vi "Main.vi"() -> ()   [LabVIEW 2022 SP3]
doc: "Use this template to build a simple state machine design pattern. Each state executes code and determines which state to transition to."
uses:
  controls/UI Data.ctl
  controls/State.ctl
  <vilib>/Utility/file.llb/Write Delimited Spreadsheet (string).vi
  <vilib>/Analysis/NI_AALBase.lvlib
panel:
  out "Zmerene vysledky":string[][](table)=[["0", "10000", "99998", "0", "99920", "0"], ["0", "0", "0", "0", "0", "0"], ["2", "10000", "99998", "0", "99920", "0"], ["0", "0", "0", "0", "0", "0"], ["0", "0", "0", "0", "0", "0"]]
  in  "Nazev souboru k ulozeni":path=path "data.txt"
  in  "Generator read error":bool
  in  "Counter read error":bool
  in  "Osciloscope read error":bool
  out "Terminal":string="RIGOL TECHNOLOGIES,DS2102A,DS2D271700283,00.03.06\nHEWLETT-PACKARD,53131A,0,3427\nAgilent Technologies,33220A,MY43002402,1.05-1.05-22-1\n+9.999795427E+004\n9.992007e+04\n+9.999795443E+004\n9.992007e+04\n+9.999795356E+004\n9.992007e+04\n+9.999795499E+004\n9.992007e+04\n+9.999795703E+004\n9.992007e+04\n+9.999795620E+004\n9.992007e+04\n"
  in  "Stop":bool
  in  "Generator source":refnum<visa-resource-name>="USB0::0x0957::0x0407::MY43002402::INSTR"
  in  "Counter source":refnum<visa-resource-name>="GPIB0::15::INSTR"
  in  "Osciloscope source":refnum<visa-resource-name>="osc"
  out "Mereni":bool
  in  "Start":bool
  in  "Nastaveni citace":T1
  in  "Pocet opakovani":u8=3 min=1 max=20
  in  "Kalibracni body":T2(array[cluster])=[{"Kmitocet"=enum."100 kHz", "Vrms (V)"=0.6}, {"Kmitocet"=enum."prazdne", "Vrms (V)"=0.6}, {"Kmitocet"=enum."100 kHz", "Vrms (V)"=2.0}, {"Kmitocet"=enum."prazdne", "Vrms (V)"=1.0}, {"Kmitocet"=enum."prazdne", "Vrms (V)"=0.6}] {"Vrms (V)" min=0.014 max=2.83}
  in  "Data":T3={"Oscilosope source"="", "Counter source"="", "Generator source"="", "Measuring?"=FALSE, "j(sample)"=0, "i(point)"=0, "Kalibracni body"=[], "Pocet opakovani"=1, "Nastaveni citace"={"Vazba"=enum."DC", "Vstupni impedance"=enum."1 MOhm", "Filtr 100 kHz"=FALSE}, "Config delay counter"=0, "GlobalState"=enum."WAITING", "Terminal"="", "namerene hodnoty osciloskop"=[], "namerene hodnoty citac"=[], "nejistoty osciloskop"=[], "nejistoty citac"=[], "vysledek citac"=[], "vysledek osciloskop"=[], "tabulka"=[]} {"Pocet opakovani" min=1 max=20}
  in  "Exit":bool
  # "Komunikace s mericimi pristroji"
  # "Spousteni mereni"
  # "Indikace stavu"
  # "Nastaveni mereni"
  # "Ne"
  # "Ano"
  # "Ano"
  # "Ne"
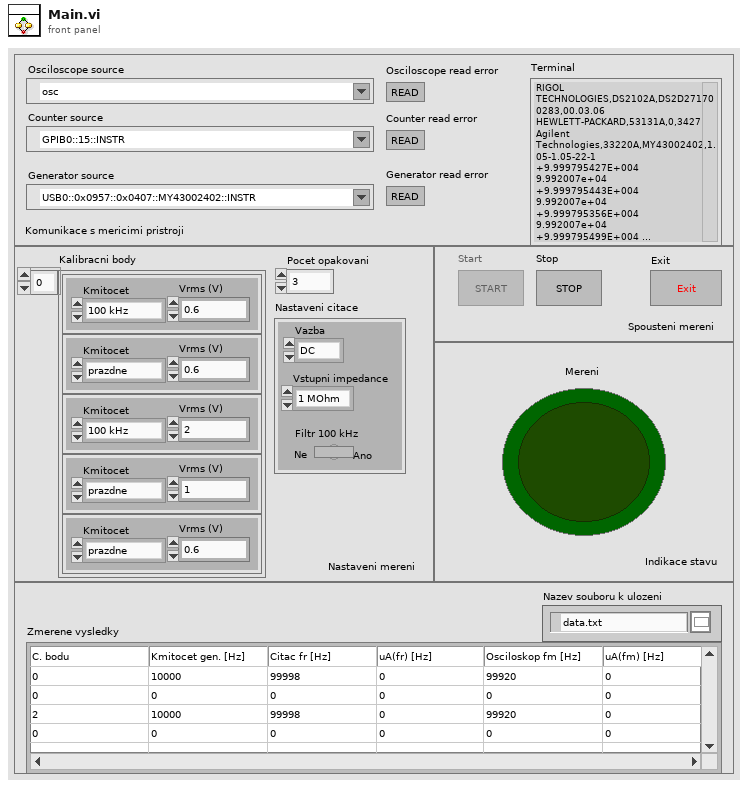
[diagram p1: front panel]
types:
  T1 = cluster{"Vazba":enum16{"DC", "AC"}, "Vstupni impedance":enum16{"1 MOhm", "50 Ohm"}, "Filtr 100 kHz":bool}
  T2 = cluster{"Kmitocet":enum16{"prazdne", "50 Hz", "1 kHz", "5 kHz", "10 kHz", "20 kHz", "50 kHz", "100 kHz"}, "Vrms (V)":dbl}[]
  T3 = typedef "UI Data.ctl" = cluster{"Oscilosope source":refnum<visa-resource-name>, "Counter source":refnum<visa-resource-name>, "Generator source":refnum<visa-resource-name>, "Measuring?":bool, "j(sample)":u8, "i(point)":u8, "Kalibracni body":cluster{"Kmitocet":enum16{"prazdne", "50 Hz", "1 kHz", "5 kHz", "10 kHz", "20 kHz", "50 kHz", "100 kHz"}, "Vrms (V)":dbl}[], "Pocet opakovani":u8, "Nastaveni citace":cluster{"Vazba":enum16{"DC", "AC"}, "Vstupni impedance":enum16{"1 MOhm", "50 Ohm"}, "Filtr 100 kHz":bool}, "Config delay counter":u8, "GlobalState":enum16{"WAITING", "NEXT", "MEASURE"}, "Terminal":string, "namerene hodnoty osciloskop":dbl[][], "namerene hodnoty citac":dbl[][], "nejistoty osciloskop":dbl[], "nejistoty citac":dbl[], "vysledek citac":dbl[], "vysledek osciloskop":dbl[], "tabulka":string[][]}
  T4 = typedef "State.ctl" = enum16{"Initialize", "Wait for Event", "Config", "Meas", "Calculate", "End meas", "Store & update", "Exit"}
  T5 = enum8{"Enabled", "Disabled", "Disabled and Grayed Out"}
  T6 = enum16{"prazdne", "50 Hz", "1 kHz", "5 kHz", "10 kHz", "20 kHz", "50 kHz", "100 kHz"}
  T7 = cluster{"Kmitocet":enum16{"prazdne", "50 Hz", "1 kHz", "5 kHz", "10 kHz", "20 kHz", "50 kHz", "100 kHz"}, "Vrms (V)":dbl}
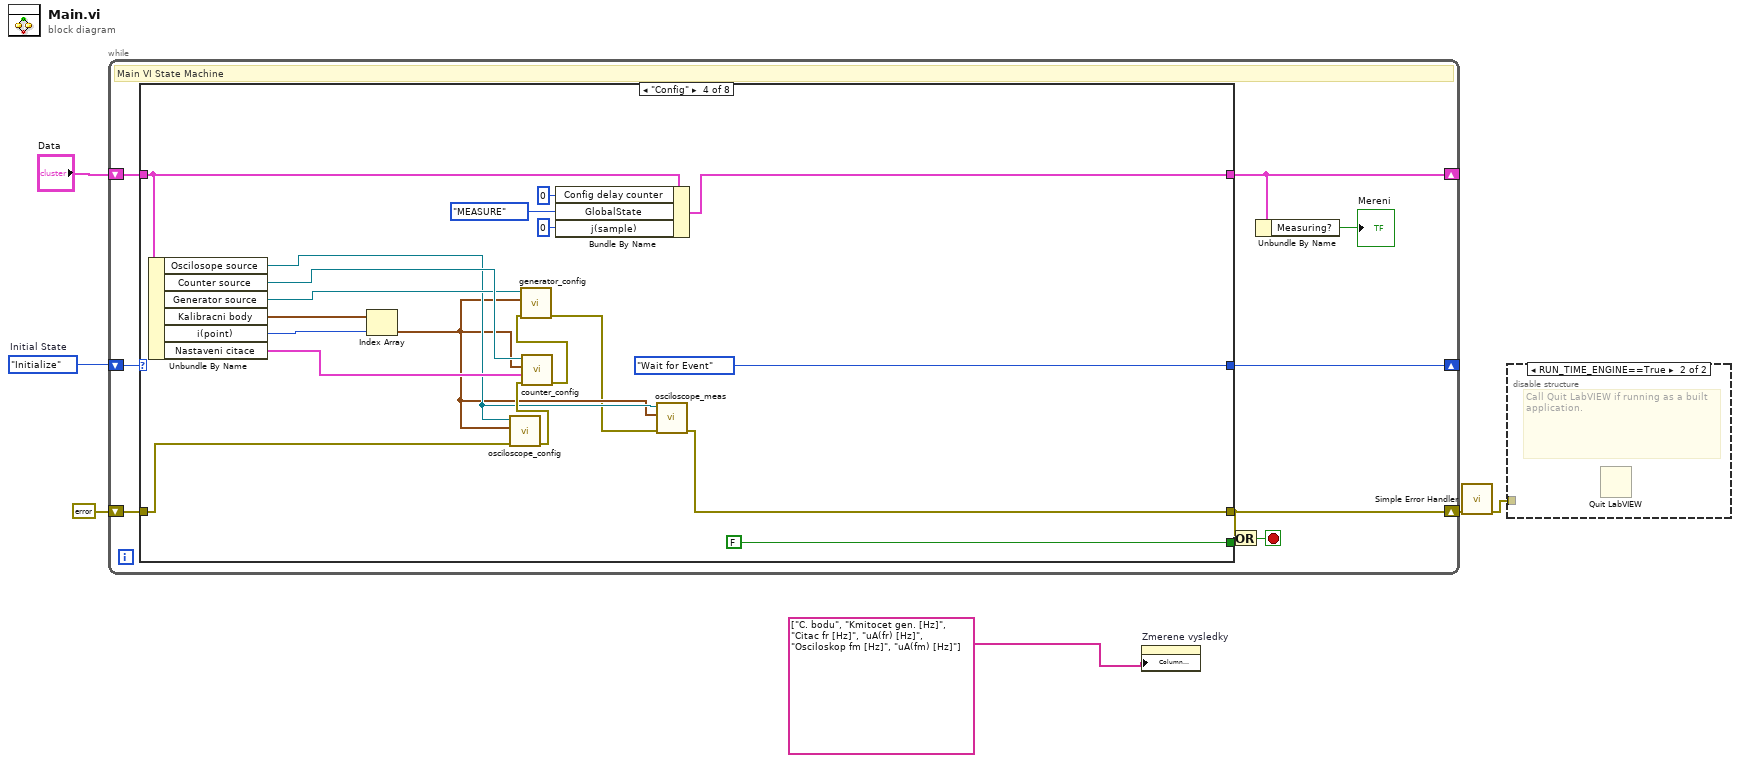
[diagram p0: block diagram]
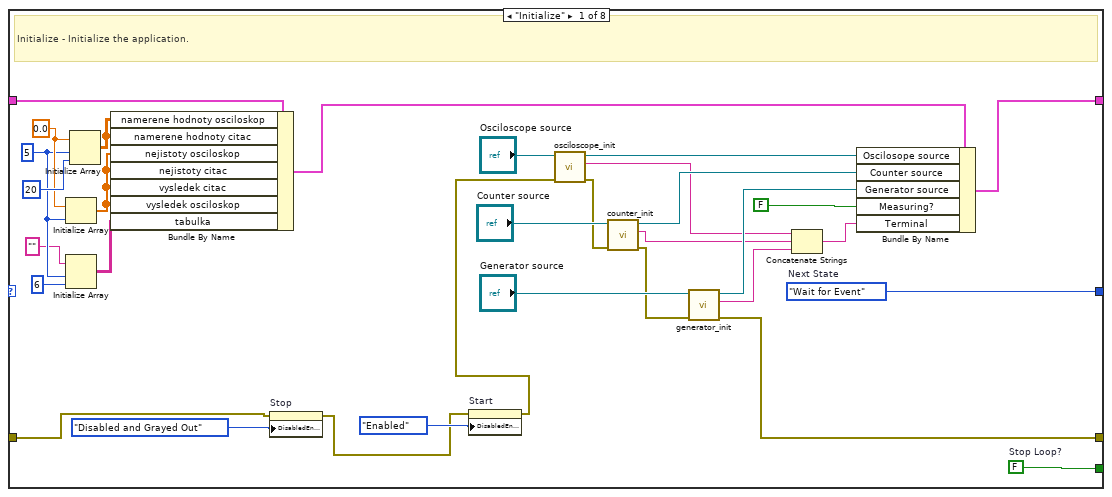
[diagram p3: hidden frame]
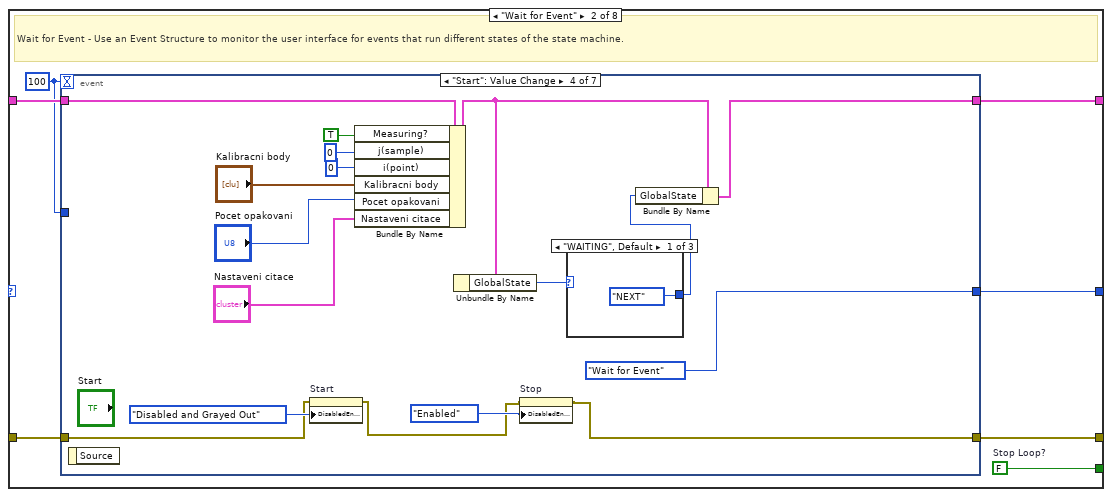
[diagram p4: hidden frame]
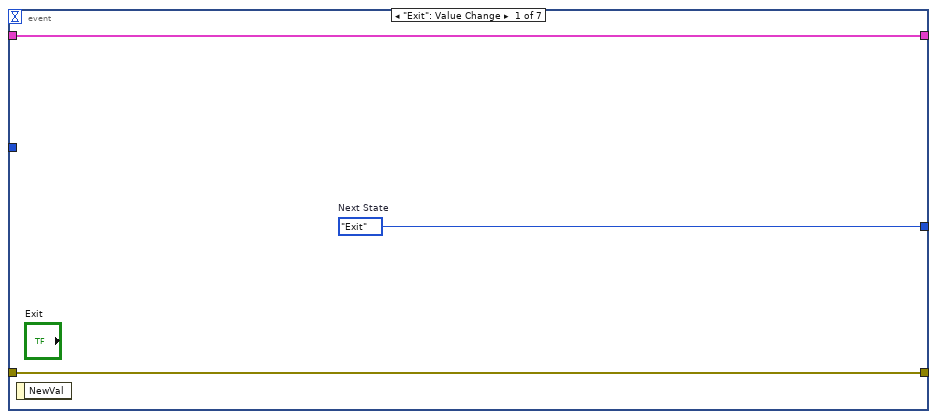
[diagram p5: hidden frame]
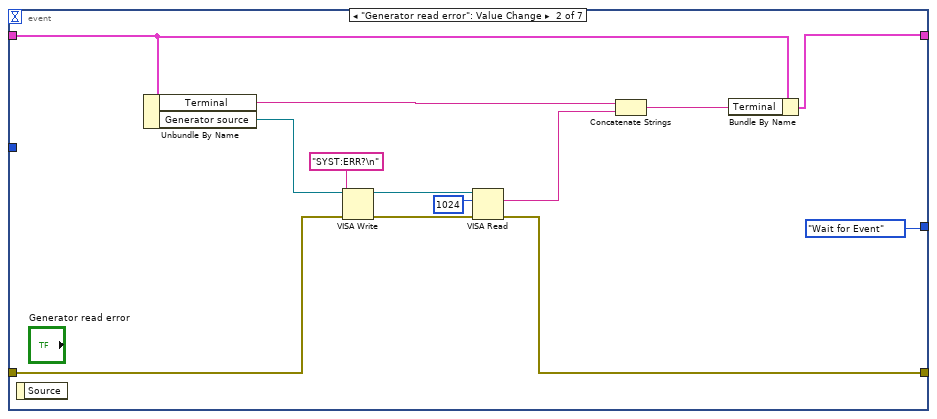
[diagram p6: hidden frame]
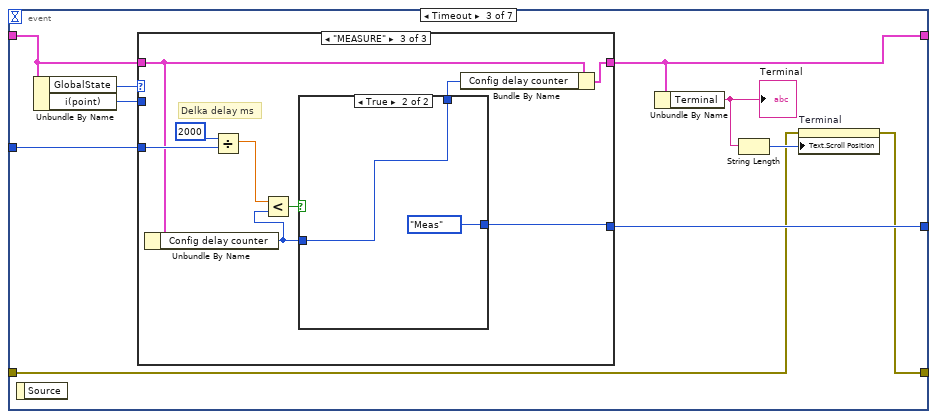
[diagram p7: hidden frame]
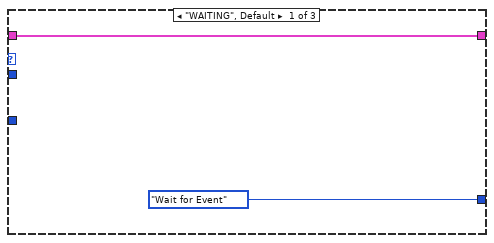
[diagram p8: hidden frame]
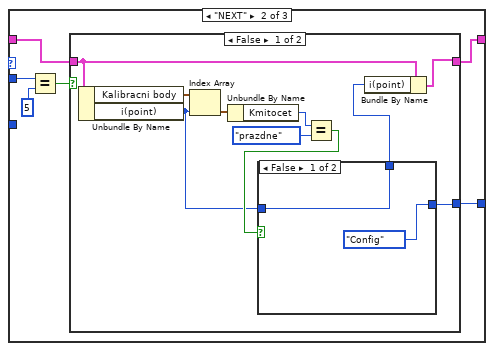
[diagram p9: hidden frame]
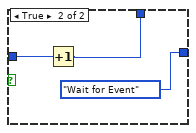
[diagram p10: hidden frame]
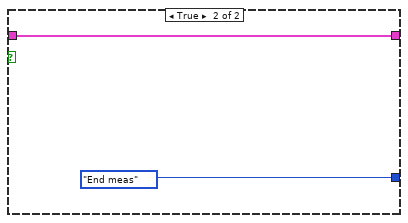
[diagram p11: hidden frame]
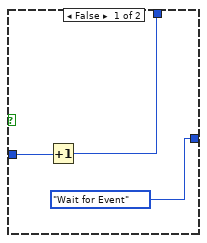
[diagram p12: hidden frame]
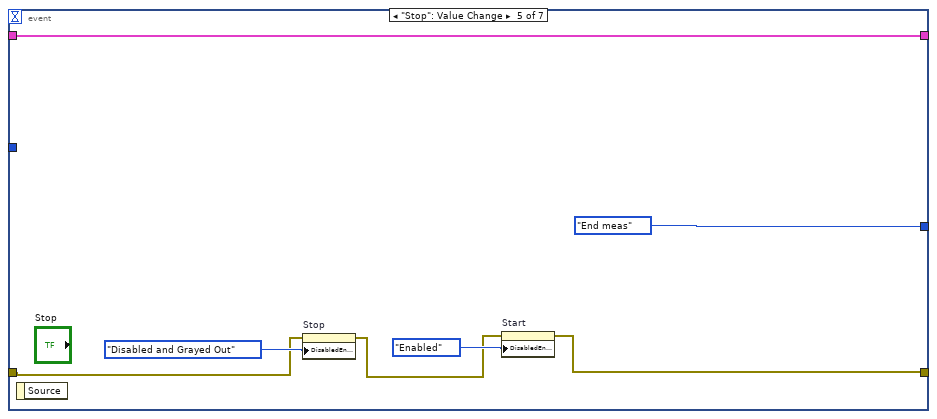
[diagram p15: hidden frame]
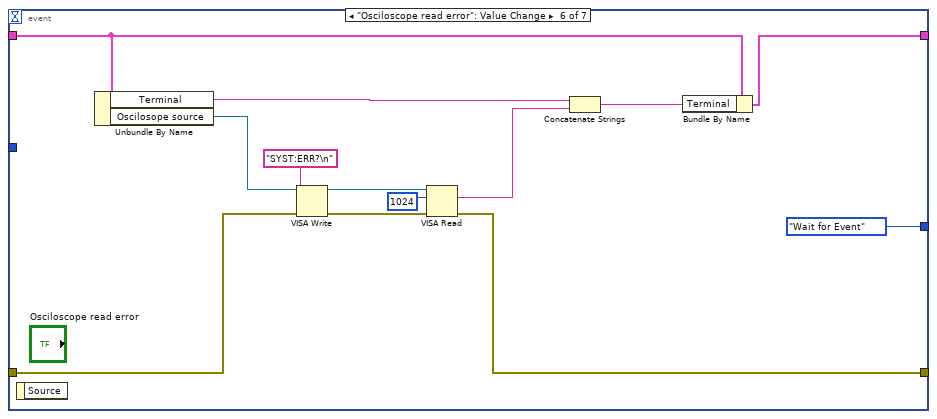
[diagram p16: hidden frame]
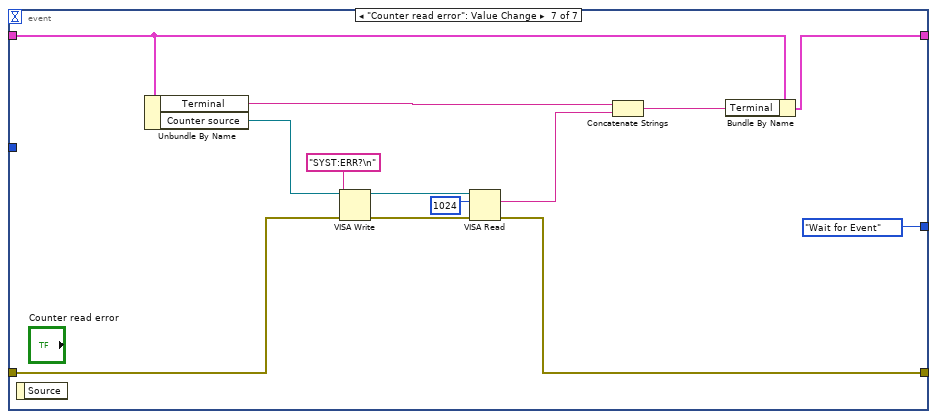
[diagram p17: hidden frame]
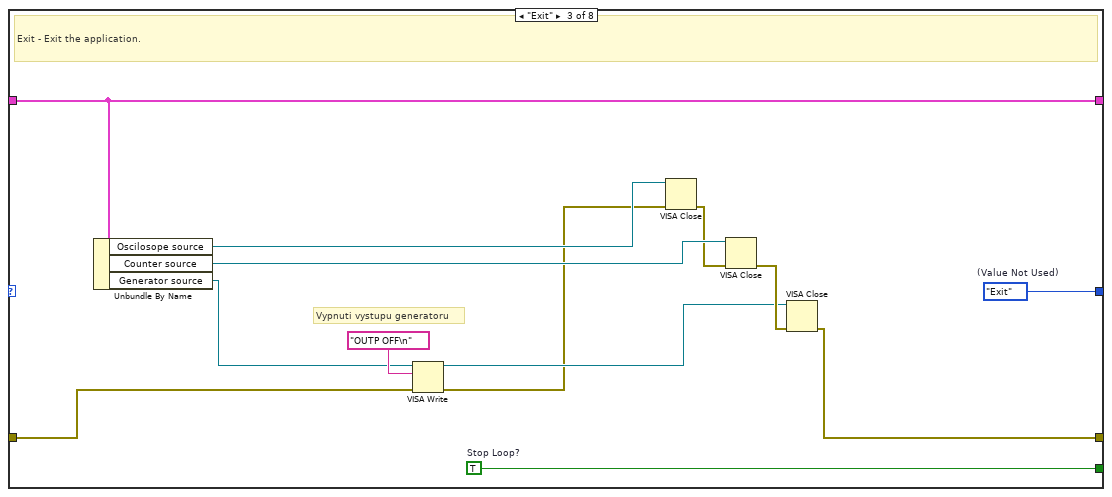
[diagram p18: hidden frame]
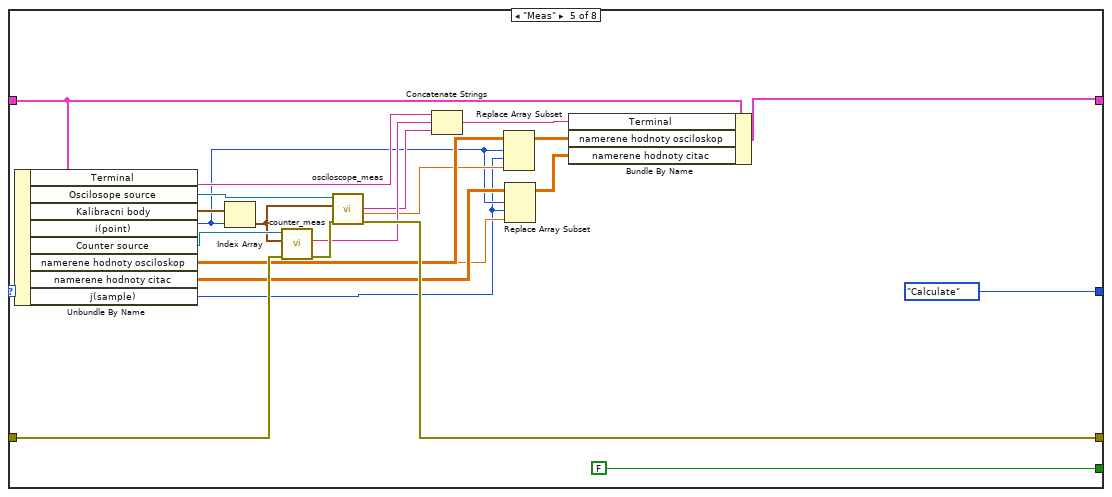
[diagram p19: hidden frame]
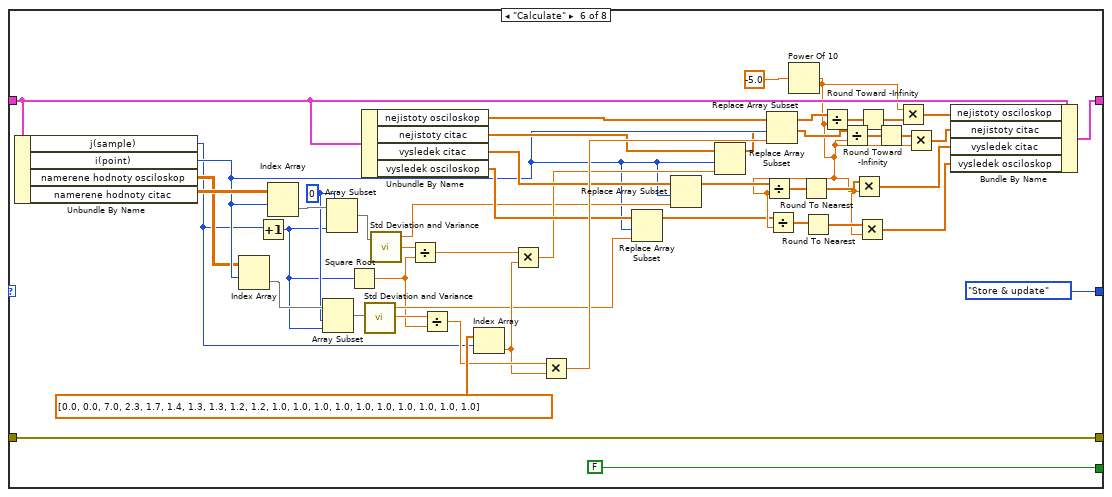
[diagram p20: hidden frame]
diagram:
  w6 = State."Initialize"  # Initial State
  n1 = while {
    shift-right: [w14] -> _
    shift-left: w6 -> [w15]
    shift-right: [w8] -> _
    shift-left: "Data" -> [w13]
    shift-right: [w9] -> w4
    shift-left: errorcluster {"status"=FALSE, "code"=0, "source"=""} ("error constant") -> [w12]
    stop <- w10 stop-if-true
    # "Main VI State Machine"
    n2 = case shown="\"Config\"" w15 {
      tunnel: [w47 w54 w185 State."Wait for Event" ("(Value Not Used)") State."Calculate" ("(Value Not Used)") State."Store & update" ("(Value Not Used)") State."Wait for Event" ("(Value Not Used)") State."Wait for Event" ("(Value Not Used)")] -> w14
      tunnel: [w46 w53 w184 FALSE ("Stop Loop?") FALSE ("Stop Loop?") FALSE ("Stop Loop?") FALSE ("Stop Loop?") FALSE ("Stop Loop?")] -> w11
      tunnel: w13 -> [w25 w52 w183 w194 w218 w266 w298 w319]
      tunnel: [w45 w51 w183 w193 w213 w265 w297 w327] -> w8
      tunnel: w12 -> [w27 w50 w174 w197 w222 w275 w301 w316]
      tunnel: [w43 w49 w178 w186 w224 w275 w301 w320] -> w9
      frame "Initialize" {
        w20 = 0.0 ("element")
        w19 = 5 ("dimension size")
        w46 = FALSE  # Stop Loop?
        w47 = State."Wait for Event"  # Next State
        # "Initialize - Initialize the application."
        n3 = Initialize Array(w20, w19) -> (w21:dbl[])
        n4 = Initialize Array("", w19, 6 ("dimension size")) -> (w17:string[][])
        n5 = Initialize Array(w20, w19, 20 ("dimension size")) -> (w23:dbl[][])
        n6 = Bundle By Name(cluster=w25, "namerene hodnoty osciloskop"=w23, "namerene hodnoty citac"=w23, "nejistoty osciloskop"=w21, "nejistoty citac"=w21, "vysledek citac"=w21, "vysledek osciloskop"=w21, "tabulka"=w17) -> (w24:T3)
        n7 = property on="Stop" class="Bool"(error in=w27, "DisabledEnum"=T5."Disabled and Grayed Out" ("Disabled")) -> (error out=w28:errorcluster)  [unwired: 1 in, 1 out]
        n8 = property on="Start" class="Bool"(error in=w28, "DisabledEnum"=T5."Enabled" ("Disabled")) -> (error out=w26:errorcluster)  [unwired: 1 in, 1 out]
        n9 = call "osciloscope_init.vi"("error in (no error)"=w26, "VISA Refnum in"="Osciloscope source") -> ("error out"=w38:errorcluster, "Raw data"=w32:string, "VISA Refnum out"=w36:refnum<visa-resource-name>)  [unwired: 7 in]
        n10 = call "counter_init.vi"("error in (no error)"=w38, "VISA Refnum in"="Counter source") -> ("error out"=w37:errorcluster, "Raw data"=w33:string, "VISA Refnum out"=w35:refnum<visa-resource-name>)  [unwired: 7 in]
        n11 = call "generator_init.vi"("error in (no error)"=w37, "VISA Refnum in"="Generator source") -> ("error out"=w43:errorcluster, "Raw data"=w34:string, "VISA Refnum out"=w42:refnum<visa-resource-name>)  [unwired: 7 in]
        n12 = Concatenate Strings(w32, w33, w34) -> (w31:string)
        n13 = Bundle By Name(cluster=w24, "Oscilosope source"=w36, "Counter source"=w35, "Generator source"=w42, "Measuring?"=FALSE, "Terminal"=w31) -> (w45:T3)
      }
      frame "Wait for Event" {
        w48 = 100
        w53 = FALSE  # Stop Loop?
        # "Wait for Event - Use an Event Structure to monitor the user interface for events that run different states of the state machine."
        n14 = event shown="[3] \"Start\": Value Change" {
          selector: _ -> [_ _ _ _ _ _ _]
          dyn-events: _ -> [_ _ _ _ _ _ _]
          timeout: w48 -> [_ _ _ _ _ _ _]
          tunnel: [w57 State."Wait for Event" ("Next State") w78 State."Wait for Event" ("Next State") State."End meas" ("Next State") State."Wait for Event" ("Next State") State."Wait for Event" ("Next State")] -> w54
          tunnel: w52 -> [w56 w62 w79 w136 w146 w150 w164]
          tunnel: [w56 w61 w75 w126 w146 w149 w163] -> w51
          tunnel: w50 -> [w55 w60 w72 w122 w142 w154 w162]
          tunnel: [w55 w59 w71 w120 w140 w153 w161] -> w49
          tunnel: w48 -> [_ _ w76 _ _ _ _]
          event "Exit": Value Change {
            w57 = State."Exit"  # Next State
            n15 = event-data() -> ()  [unwired: 1 in, 1 out]
          }
          event "Generator read error": Value Change {
            n16 = event-data() -> ()  [unwired: 1 in, 1 out]
            n17 = Unbundle By Name(w62) -> ("Terminal"=w65:string, "Generator source"=w66:refnum<visa-resource-name>)
            n18 = VISA Write(VISA resource name=w66, write buffer="SYST:ERR?\n", error in (no error)=w60) -> (VISA resource name out=w69:refnum<visa-resource-name>, error out=w68:errorcluster)  [unwired: 1 out]
            n19 = VISA Read(VISA resource name=w69, byte count=u32 1024, error in (no error)=w68) -> (read buffer=w64:string, error out=w59:errorcluster)  [unwired: 2 out]
            n20 = Concatenate Strings(w65, w64) -> (w63:string)
            n21 = Bundle By Name(cluster=w62, "Terminal"=w63) -> (w61:T3)
          }
          event Timeout {
            n22 = event-data() -> ()  [unwired: 1 in, 1 out]
            n23 = Unbundle By Name(w79) -> ("GlobalState"=w80:enum16{"WAITING", "NEXT", "MEASURE"}, "i(point)"=w77:u8)
            n24 = case shown="\"MEASURE\"" w80 {
              tunnel: w79 -> [w82 w84 w109]
              tunnel: [w82 w83 w106] -> w75
              tunnel: [State."Wait for Event" ("Next State") w85 w110] -> w78
              tunnel: w77 -> [_ w87 _]
              tunnel: w76 -> [_ _ w114]
              frame "WAITING", Default {
              }
              frame "NEXT" {
                n25 = Equal?(x=w87, y=u8 5) -> (x = y?=w88:bool)
                n26 = case shown="False" w88 {
                  tunnel: [w89 State."End meas" ("Next State")] -> w85
                  tunnel: w84 -> [w92 w104]
                  tunnel: [w90 w104] -> w83
                  frame False {
                    n27 = Unbundle By Name(w92) -> ("Kalibracni body"=w98:T2, "i(point)"=w93:u8)
                    n28 = Index Array(array=w98, index=w93) -> (element=w97:T7)
                    n29 = Unbundle By Name(w97) -> ("Kmitocet"=w95:T6)
                    n30 = Equal?(x=w95, y=T6."prazdne") -> (x = y?=w94:bool)
                    n31 = case shown="False" w94 {
                      tunnel: w93 -> [w100 w103]
                      tunnel: [w100 w102] -> w91
                      tunnel: [State."Config" ("Next State") State."Wait for Event" ("Next State")] -> w89
                      frame False {
                      }
                      frame True {
                        n32 = Increment(x=w103) -> (x+1=w102:u8)
                      }
                    }
                    n33 = Bundle By Name(cluster=w92, "i(point)"=w91) -> (w90:T3)
                  }
                  frame True {
                  }
                }
              }
              frame "MEASURE" {
                # "Delka delay ms"
                n34 = Unbundle By Name(w109) -> ("Config delay counter"=w108:u8)
                n35 = Divide(x=2000, y=w114) -> (x/y=w111:dbl)
                n36 = Less?(x=w111, y=w108) -> (x < y?=w112:bool)
                n37 = case shown="True" w112 {
                  tunnel: [State."Wait for Event" ("Next State") State."Meas" ("Next State")] -> w110
                  tunnel: w108 -> [w117 w118]
                  tunnel: [w116 w118] -> w107
                  frame False {
                    n38 = Increment(x=w117) -> (x+1=w116:u8)
                  }
                  frame True {
                  }
                }
                n39 = Bundle By Name(cluster=w109, "Config delay counter"=w107) -> (w106:T3)
              }
            }
            n40 = Unbundle By Name(w75) -> ("Terminal"=w74:string)
            "Terminal" <- w74
            n41 = String Length(string=w74) -> (length=w73:i32)
            n42 = property on="Terminal" class="Str"(error in=w72, "Text.Scroll Position"=w73) -> (error out=w71:errorcluster)  [unwired: 1 in, 1 out]
          }
          event "Start": Value Change {
            n43 = event-data() -> ()  [unwired: 1 in, 1 out]
            n44 = property on="Start" class="Bool"(error in=w122, "DisabledEnum"=T5."Disabled and Grayed Out" ("Disabled")) -> (error out=w121:errorcluster)  [unwired: 1 in, 1 out]
            n45 = Bundle By Name(cluster=w136, "Measuring?"=TRUE, "j(sample)"=u8 0, "i(point)"=u8 0, "Kalibracni body"="Kalibracni body", "Pocet opakovani"="Pocet opakovani", "Nastaveni citace"="Nastaveni citace") -> (w127:T3)
            n46 = Unbundle By Name(w127) -> ("GlobalState"=w129:enum16{"WAITING", "NEXT", "MEASURE"})
            n47 = property on="Stop" class="Bool"(error in=w121, "DisabledEnum"=T5."Enabled" ("Disabled")) -> (error out=w120:errorcluster)  [unwired: 1 in, 1 out]
            n48 = case shown="\"WAITING\", Default" w129 {
              selector: w129 -> [_ w138 w139]
              tunnel: [enum16{"WAITING", "NEXT", "MEASURE"}."NEXT" ("GlobalState") w138 w139] -> w125
              frame "WAITING", Default {
              }
              frame "NEXT" {
              }
              frame "MEASURE" {
              }
            }
            n49 = Bundle By Name(cluster=w127, "GlobalState"=w125) -> (w126:T3)
          }
          event "Stop": Value Change {
            n50 = event-data() -> ()  [unwired: 1 in, 1 out]
            n51 = property on="Stop" class="Bool"(error in=w142, "DisabledEnum"=T5."Disabled and Grayed Out" ("Disabled")) -> (error out=w141:errorcluster)  [unwired: 1 in, 1 out]
            n52 = property on="Start" class="Bool"(error in=w141, "DisabledEnum"=T5."Enabled" ("Disabled")) -> (error out=w140:errorcluster)  [unwired: 1 in, 1 out]
          }
          event "Osciloscope read error": Value Change {
            n53 = event-data() -> ()  [unwired: 1 in, 1 out]
            n54 = Unbundle By Name(w150) -> ("Terminal"=w152:string, "Oscilosope source"=w155:refnum<visa-resource-name>)
            n55 = VISA Write(VISA resource name=w155, write buffer="SYST:ERR?\n", error in (no error)=w154) -> (VISA resource name out=w158:refnum<visa-resource-name>, error out=w157:errorcluster)  [unwired: 1 out]
            n56 = VISA Read(VISA resource name=w158, byte count=u32 1024, error in (no error)=w157) -> (read buffer=w151:string, error out=w153:errorcluster)  [unwired: 2 out]
            n57 = Concatenate Strings(w152, w151) -> (w148:string)
            n58 = Bundle By Name(cluster=w150, "Terminal"=w148) -> (w149:T3)
          }
          event "Counter read error": Value Change {
            n59 = event-data() -> ()  [unwired: 1 in, 1 out]
            n60 = Unbundle By Name(w164) -> ("Terminal"=w167:string, "Counter source"=w168:refnum<visa-resource-name>)
            n61 = VISA Write(VISA resource name=w168, write buffer="SYST:ERR?\n", error in (no error)=w162) -> (VISA resource name out=w171:refnum<visa-resource-name>, error out=w170:errorcluster)  [unwired: 1 out]
            n62 = VISA Read(VISA resource name=w171, byte count=u32 1024, error in (no error)=w170) -> (read buffer=w166:string, error out=w161:errorcluster)  [unwired: 2 out]
            n63 = Concatenate Strings(w167, w166) -> (w165:string)
            n64 = Bundle By Name(cluster=w164, "Terminal"=w165) -> (w163:T3)
          }
        }
      }
      frame "Exit" {
        w184 = TRUE  # Stop Loop?
        w185 = State."Exit"  # (Value Not Used)
        # "Vypnuti vystupu generatoru"
        # "Exit - Exit the application."
        n65 = Unbundle By Name(w183) -> ("Oscilosope source"=w182:refnum<visa-resource-name>, "Counter source"=w181:refnum<visa-resource-name>, "Generator source"=w176:refnum<visa-resource-name>)
        n66 = VISA Write(VISA resource name=w176, write buffer="OUTP OFF\n", error in (no error)=w174) -> (VISA resource name out=w175:refnum<visa-resource-name>, error out=w173:errorcluster)  [unwired: 1 out]
        n67 = VISA Close(VISA resource name=w182, error in (no error)=w173) -> (error out=w180:errorcluster)
        n68 = VISA Close(VISA resource name=w181, error in (no error)=w180) -> (error out=w179:errorcluster)
        n69 = VISA Close(VISA resource name=w175, error in (no error)=w179) -> (error out=w178:errorcluster)
      }
      frame "Config" {
        n70 = Unbundle By Name(w194) -> ("Oscilosope source"=w189:refnum<visa-resource-name>, "Counter source"=w202:refnum<visa-resource-name>, "Generator source"=w201:refnum<visa-resource-name>, "Kalibracni body"=w199:T2, "i(point)"=w198:u8, "Nastaveni citace"=w200:T1)
        n71 = Index Array(array=w199, index=w198) -> (element=w188:T7)
        n72 = call "osciloscope_config.vi"("error in (no error)"=w197, "Kalibracni bod"=w188, "VISA Refnum in"=w189) -> ("error out"=w196:errorcluster)  [unwired: 7 in, 1 out]
        n73 = call "counter_config.vi"("error in (no error)"=w196, "Nastaveni citace"=w200, "Kalibracni bod"=w188, "VISA Refnum in"=w202) -> ("error out"=w195:errorcluster)  [unwired: 6 in, 1 out]
        n74 = call "generator_config.vi"("error in (no error)"=w195, "Kalibracni bod"=w188, "VISA Refnum in"=w201) -> ("error out"=w187:errorcluster)  [unwired: 7 in, 1 out]
        n75 = Bundle By Name(cluster=w194, "Config delay counter"=u8 0, "GlobalState"=enum16{"WAITING", "NEXT", "MEASURE"}."MEASURE", "j(sample)"=u8 0) -> (w193:T3)
        n76 = call "osciloscope_meas.vi"("error in (no error)"=w187, "Kalibracni bod"=w188, "VISA Refnum in"=w189) -> ("error out"=w186:errorcluster)  [unwired: 4 in, 3 out]
      }
      frame "Meas" {
        n77 = Unbundle By Name(w218) -> ("Terminal"=w217:string, "Oscilosope source"=w225:refnum<visa-resource-name>, "Kalibracni body"=w220:T2, "i(point)"=w206:u8, "Counter source"=w221:refnum<visa-resource-name>, "namerene hodnoty osciloskop"=w212:dbl[][], "namerene hodnoty citac"=w209:dbl[][], "j(sample)"=w205:u8)
        n78 = Index Array(array=w220, index=w206) -> (element=w219:T7)
        n79 = call "counter_meas.vi"("error in (no error)"=w222, "Kalibracni bod"=w219, "VISA Refnum in"=w221) -> ("error out"=w223:errorcluster, "number"=w207:dbl, "Raw data"=w216:string)  [unwired: 4 in, 1 out]
        n80 = call "osciloscope_meas.vi"("error in (no error)"=w223, "Kalibracni bod"=w219, "VISA Refnum in"=w225) -> ("error out"=w224:errorcluster, "number"=w211:dbl, "Raw data"=w215:string)  [unwired: 4 in, 1 out]
        n81 = Concatenate Strings(w217, w216, w215) -> (w214:string)
        n82 = Replace Array Subset(array=w212, new element=w211, index (row)=w206, index (col)=w205) -> (w210:dbl[][])
        n83 = Replace Array Subset(array=w209, new element=w207, index (row)=w206, index (col)=w205) -> (w208:dbl[][])
        n84 = Bundle By Name(cluster=w218, "Terminal"=w214, "namerene hodnoty osciloskop"=w210, "namerene hodnoty citac"=w208) -> (w213:T3)
      }
      frame "Calculate" {
        w248 = 0 ("index")
        n85 = Unbundle By Name(w266) -> ("j(sample)"=w249:u8, "i(point)"=w255:u8, "namerene hodnoty osciloskop"=w254:dbl[][], "namerene hodnoty citac"=w270:dbl[][])
        n86 = Index Array(array=w254, index (row)=w255) -> (element=w253:dbl[])  [unwired: 1 in]
        n87 = Increment(x=w249) -> (x+1=w247:u8)
        n88 = Index Array(array=w270, index (row)=w255) -> (element=w252:dbl[])  [unwired: 1 in]
        n89 = Array Subset(array=w253, index=w248, length=w247) -> (w250:dbl[])
        n90 = Array Subset(array=w252, index=w248, length=w247) -> (w251:dbl[])
        n91 = Square Root(x=w247) -> (sqrt(x)=w246:dbl)
        n92 = Unbundle By Name(w266) -> ("nejistoty osciloskop"=w267:dbl[], "nejistoty citac"=w263:dbl[], "vysledek citac"=w262:dbl[], "vysledek osciloskop"=w261:dbl[])
        n93 = call <vilib>:"Std Deviation and Variance.vi"("X"=w250) -> ("mean"=w256:dbl, "standard deviation"=w257:dbl)  [unwired: 1 in, 1 out]
        n94 = call <vilib>:"Std Deviation and Variance.vi"("X"=w251) -> ("mean"=w258:dbl, "standard deviation"=w259:dbl)  [unwired: 1 in, 1 out]
        n95 = Divide(x=w259, y=w246) -> (x/y=w269:dbl)
        n96 = Divide(x=w257, y=w246) -> (x/y=w271:dbl)
        n97 = Index Array(array=dbl[] [0.0, 0.0, 7.0, 2.3, 1.7, 1.4, 1.3, 1.3, 1.2, 1.2, 1.0, 1.0, 1.0, 1.0, 1.0, 1.0, 1.0, 1.0, 1.0, 1.0], index=w249) -> (element=w268:dbl)
        n98 = Multiply(x=w269, y=w268) -> (x*y=w260:dbl)
        n99 = Multiply(x=w271, y=w268) -> (x*y=w264:dbl)
        n100 = Replace Array Subset(array=w261, new element=w256, index=w255) -> (w229:dbl[])
        n101 = Replace Array Subset(array=w262, new element=w258, index=w255) -> (w234:dbl[])
        n102 = Replace Array Subset(array=w263, new element=w260, index=w255) -> (w237:dbl[])
        n103 = Replace Array Subset(array=w267, new element=w264, index=w255) -> (w241:dbl[])
        n104 = Power Of 10(x=-5.0) -> (10^x=w230:dbl)
        n105 = Divide(x=w234, y=w230) -> (x/y=w235:dbl[])
        n106 = Divide(x=w229, y=w230) -> (x/y=w232:dbl[])
        n107 = Round To Nearest(number=w235) -> (nearest integer value=w236:dbl[])
        n108 = Round To Nearest(number=w232) -> (nearest integer value=w231:dbl[])
        n109 = Divide(x=w241, y=w230) -> (x/y=w242:dbl[])
        n110 = Divide(x=w237, y=w230) -> (x/y=w245:dbl[])
        n111 = Multiply(x=w236, y=w230) -> (x*y=w233:dbl[])
        n112 = Multiply(x=w231, y=w230) -> (x*y=w228:dbl[])
        n113 = Round Toward -Infinity(1:w242) -> (0:w238:dbl[])
        n114 = Round Toward -Infinity(1:w245) -> (0:w244:dbl[])
        n115 = Multiply(x=w230, y=w238) -> (x*y=w240:dbl[])
        n116 = Multiply(x=w244, y=w230) -> (x*y=w243:dbl[])
        n117 = Bundle By Name(cluster=w266, "nejistoty osciloskop"=w240, "nejistoty citac"=w243, "vysledek citac"=w233, "vysledek osciloskop"=w228) -> (w265:T3)
      }
      frame "Store & update" {
        n118 = Unbundle By Name(w298) -> ("j(sample)"=w299:u8, "Pocet opakovani"=w294:u8, "i(point)"=w283:u8, "vysledek citac"=w281:dbl[], "nejistoty citac"=w280:dbl[], "vysledek osciloskop"=w279:dbl[], "nejistoty osciloskop"=w278:dbl[], "Kalibracni body"=w288:T2, "tabulka"=w277:string[][])
        n119 = Index Array(array=w288, index=w283) -> (element=w287:T7)
        n120 = Increment(x=w299) -> (x+1=w295:u8)
        n121 = Unbundle By Name(w287) -> ("Kmitocet"=w285:T6)
        n122 = Equal?(x=w295, y=w294) -> (x = y?=w296:bool)
        n123 = case shown="True" w296 {
          tunnel: [enum16{"WAITING", "NEXT", "MEASURE"}."MEASURE" ("GlobalState") enum16{"WAITING", "NEXT", "MEASURE"}."NEXT" ("GlobalState")] -> w293
          tunnel: w283 -> [w310 w313]
          tunnel: [w310 w312] -> w292
          frame False {
          }
          frame True {
            n124 = Increment(x=w313) -> (x+1=w312:u8)
          }
        }
        n125 = case shown="\"1 kHz\"" w285 {
          tunnel: [0 50 1000 5000 10000 20000 50000 100000] -> w282
          frame "prazdne", Default {
          }
          frame "50 Hz" {
          }
          frame "1 kHz" {
          }
          frame "5 kHz" {
          }
          frame "10 kHz" {
          }
          frame "20 kHz" {
          }
          frame "50 kHz" {
          }
          frame "100 kHz" {
          }
        }
        n126 = call "table_number_stringI.vi"("nejistota osciloskop"=w278, "cislo mereni"=w283, "vysledek osciloskop"=w279, "nejistota citac"=w280, "vysledek citac"=w281, "kmitocet gen"=w282) -> ("Array"=w284:string[])  [unwired: 5 in]
        n127 = Replace Array Subset(array=w277, new element=w284, index (row)=w283) -> (w276:string[][])  [unwired: 1 in]
        "Zmerene vysledky" <- w276
        n128 = Bundle By Name(cluster=w298, "j(sample)"=w295, "GlobalState"=w293, "i(point)"=w292, "tabulka"=w276) -> (w297:T3)
        n129 = call <vilib>:"Application Directory.vi"() -> ("Application Directory"=w290:path)
        n130 = Build Path(base path=w290, name or relative path="Nazev souboru k ulozeni") -> (appended path=w289:path)
        n131 = call-poly <vilib>:"Write Delimited Spreadsheet.vi"("file path (dialog if empty)"=w289, "2D data"=w276) -> ()  [unwired: 12 in, 2 out]
      }
      frame "End meas" {
        # "Vypnuti vystupu generatoru"
        n132 = Unbundle By Name(w319) -> ("Generator source"=w318:refnum<visa-resource-name>)
        n133 = VISA Write(VISA resource name=w318, write buffer="OUTP OFF\n", error in (no error)=w316) -> (error out=w315:errorcluster)  [unwired: 2 out]
        n134 = property on="Stop" class="Bool"(error in=w315, "DisabledEnum"=T5."Disabled and Grayed Out" ("Disabled")) -> (error out=w321:errorcluster)  [unwired: 1 in, 1 out]
        n135 = property on="Start" class="Bool"(error in=w321, "DisabledEnum"=T5."Enabled" ("Disabled")) -> (error out=w320:errorcluster)  [unwired: 1 in, 1 out]
        n136 = Bundle By Name(cluster=w319, "i(point)"=u8 0, "GlobalState"=enum16{"WAITING", "NEXT", "MEASURE"}."WAITING", "Measuring?"=FALSE) -> (w327:T3)
      }
    }
    n137 = Or(x=w9, y=w11) -> (x .or. y?=w10:bool)
    n138 = Unbundle By Name(w8) -> ("Measuring?"=→"Mereni":bool)
  }
  n139 = property on="Zmerene vysledky" class="Tbl (strict)"("Column Headers[]"=string[] ["C. bodu", "Kmitocet gen. [Hz]", "Citac fr [Hz]", "uA(fr) [Hz]", "Osciloskop fm [Hz]", "uA(fm) [Hz]"] ("Column Header Strings[]")) -> ()  [unwired: 2 in, 2 out]
  n140 = call <vilib>:"Simple Error Handler.vi"("error in (no error)"=w4) -> ("error out"=w3:errorcluster)  [unwired: 4 in, 4 out]
  n141 = disable-structure shown="RUN_TIME_ENGINE==True" {
    disable-tunnel: w3 -> [_ _]
    frame condition #0 (active) {
    }
    frame condition #1 {
      # "Call Quit LabVIEW if running as a built application."
      n142 = Quit LabVIEW() -> ()  [unwired: 1 in]
    }
  }
